vi "TEA_Encrypt.vi"(8 "error in (no error)":errorcluster, 9 "k":u32[](array[numeric])=[1, 2, 3, 4], 10 "V":u32[](array[numeric])=[0, 0]) -> (0 "error out":errorcluster, 2 "Y":u32[](array[numeric]))   [LabVIEW 2009]
doc: "This VI encrypts the 64-bit number (V) using the 128-bit key (k). It returns the encrypted number (Y)."
panel:
  # "Select Help»Show Context Help and move the cursor over the VI icon to display help for this VI."
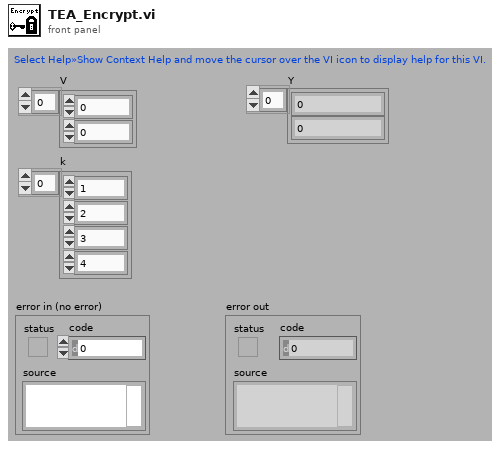
[diagram p1: front panel]
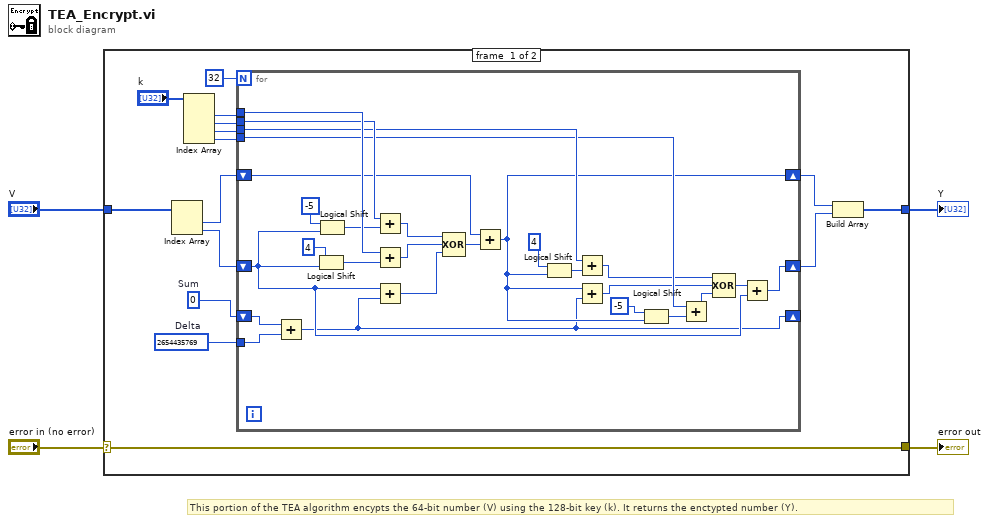
[diagram p0: block diagram]
diagram:
  # "This portion of the TEA algorithm encypts the 64-bit number (V) using the 128-bit key (k). It returns the enctypted number (Y)."
  n1 = case shown="No Error" "error in (no error)" {
    selector: "error in (no error)" -> [w7 w48]
    tunnel: [w7 w48] -> w3
    tunnel: [w6 w47] -> w2
    tunnel: "V" -> [w5 w47]
    frame #0 {
      w18 = u32 0  # Sum
      w19 = u32 2654435769  # Delta
      n2 = Index Array(array=w5) -> (element #1=w17:u32, element #2=w16:u32)  [unwired: 2 in]
      n3 = Index Array(array="k") -> (element #1=w8:u32, element #2=w14:u32, element #3=w13:u32, element #4=w12:u32)  [unwired: 4 in]
      n4 = for {
        N: 32 -> [_]
        shift-right: [w29] -> w10
        shift-left: w17 -> [w32]
        shift-right: [w30] -> w9
        shift-left: w16 -> [w31]
        shift-right: [w28] -> _
        shift-left: w18 -> [w46]
        tunnel: w19 -> [w45]
        tunnel: w8 -> [w43]
        tunnel: w14 -> [w39]
        tunnel: w13 -> [w36]
        tunnel: w12 -> [w33]
        n5 = Add(x=w46, y=w45) -> (x+y=w28:u32)
        n6 = Logical Shift(y=u32 4, x=w31) -> (x << y=w44:u32)
        n7 = Logical Shift(y=-5, x=w31) -> (x << y=w40:u32)
        n8 = Add(x=w39, y=w40) -> (x+y=w22:u32)
        n9 = Add(x=w43, y=w44) -> (x+y=w21:u32)
        n10 = Add(x=w31, y=w28) -> (x+y=w20:u32)
        n11 = Compound Arithmetic op=XOR(w22, w21, w20) -> (w27:u32)
        n12 = Add(x=w32, y=w27) -> (x+y=w29:u32)
        n13 = Logical Shift(y=u32 4, x=w29) -> (x << y=w37:u32)
        n14 = Add(x=w36, y=w37) -> (x+y=w26:u32)
        n15 = Add(x=w29, y=w28) -> (x+y=w25:u32)
        n16 = Logical Shift(y=-5, x=w29) -> (x << y=w34:u32)
        n17 = Add(x=w33, y=w34) -> (x+y=w24:u32)
        n18 = Compound Arithmetic op=XOR(w26, w25, w24) -> (w23:u32)
        n19 = Add(x=w23, y=w31) -> (x+y=w30:u32)
      }
      n20 = Build Array(w10, w9) -> (w6:u32[])
    }
    frame #1 {
    }
  }
  "error out" <- w3
  "Y" <- w2
